vi "Climber_Joystick_to_Commands.vi"(11 "Driver Inputs":T2) -> (3 "Climber_Commands":T1)   [LabVIEW 2012]
uses:
  Joystick_Inputs.ctl
  <vilib>/Rock Robotics/WPI/Joystick/WPI_JoystickButtonState.ctl
  Climber_Commands.ctl
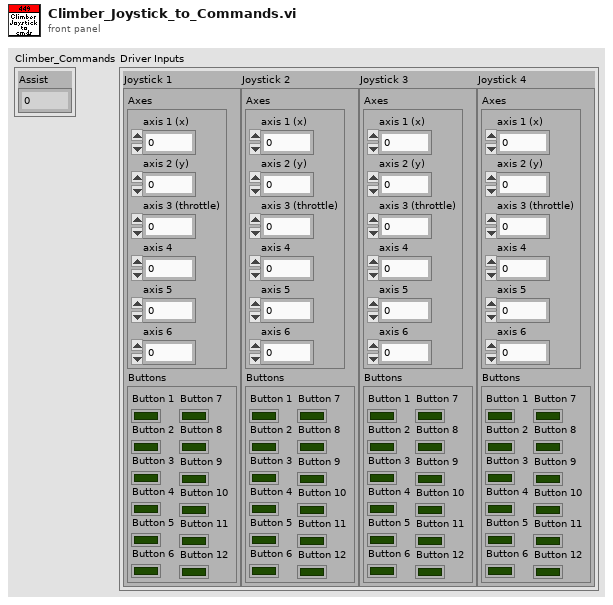
[diagram p1: front panel]
types:
  T1 = typedef "Climber_Commands.ctl" = cluster{"Assist":dbl}
  T2 = typedef "Joystick_Inputs.ctl" = cluster{"Joystick 1":cluster{"Axes":cluster{"axis 1 (x)":dbl, "axis 2 (y)":dbl, "axis 3 (throttle)":dbl, "axis 4":dbl, "axis 5":dbl, "axis 6":dbl}, "Buttons":T3}, "Joystick 2":cluster{"Axes":cluster{"axis 1 (x)":dbl, "axis 2 (y)":dbl, "axis 3 (throttle)":dbl, "axis 4":dbl, "axis 5":dbl, "axis 6":dbl}, "Buttons":T3}, "Joystick 3":cluster{"Axes":cluster{"axis 1 (x)":dbl, "axis 2 (y)":dbl, "axis 3 (throttle)":dbl, "axis 4":dbl, "axis 5":dbl, "axis 6":dbl}, "Buttons":T3}, "Joystick 4":cluster{"Axes":cluster{"axis 1 (x)":dbl, "axis 2 (y)":dbl, "axis 3 (throttle)":dbl, "axis 4":dbl, "axis 5":dbl, "axis 6":dbl}, "Buttons":T3}}
  T3 = typedef "WPI_JoystickButtonState.ctl" = cluster{"Button 1":bool, "Button 2":bool, "Button 3":bool, "Button 4":bool, "Button 5":bool, "Button 6":bool, "Button 7":bool, "Button 8":bool, "Button 9":bool, "Button 10":bool, "Button 11":bool, "Button 12":bool}
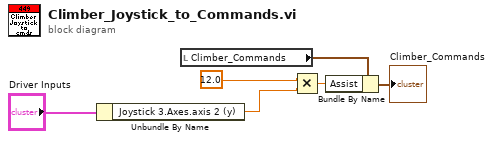
[diagram p0: block diagram]
diagram:
  n1 = Unbundle By Name("Driver Inputs") -> ("Joystick 3.Axes.axis 2 (y)"=w2:dbl)
  n2 = local read "Climber_Commands"() -> (w4:T1)
  n3 = Multiply(x=12.0 ("t"), y=w2) -> (x*y=w3:dbl)
  n4 = Bundle By Name(cluster=w4, "Assist"=w3) -> (→"Climber_Commands":T1)
